vi "myRIO_BRig_RT_dataCurrent_Tcycle_ENL.vi"() -> (2 "output_ENL":i32)   [LabVIEW 2014]
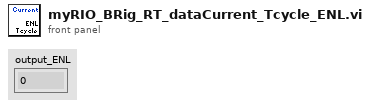
[diagram p1: front panel]
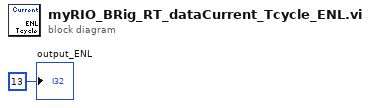
[diagram p0: block diagram]
diagram:
  "output_ENL" <- 13 ("output_iBlock")
